vi "CreateRequests.vi"(8 "error in (no error)":errorcluster) -> (0 "error out":errorcluster, 3 "StandardRequests":T1)   [LabVIEW 2024, in "Module.lvclass"]
uses:
  Module.lvclass
  Module.lvclass/Module.ctl
  StopEventArgs.ctl
  StandardRequests.ctl
  Show Front Panel--Args.ctl
  Hide Front Panel.ctl
  Show Block Diagram.ctl
  Hide Block Diagram--Args.ctl
  InitialiseArgs.ctl
  Reply.ctl
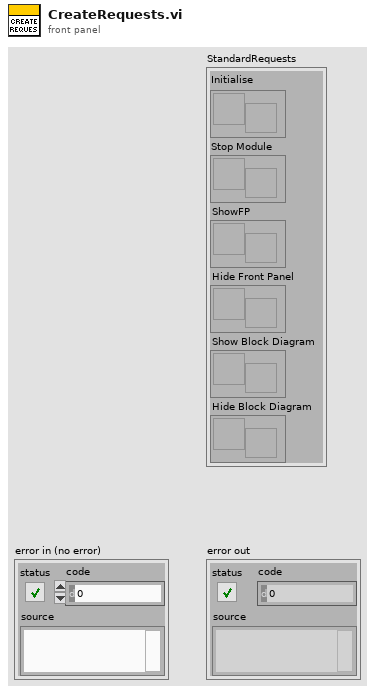
[diagram p1: front panel]
types:
  T1 = typedef "Module.lvclass/StandardRequests.ctl" = cluster{"Initialise":refnum<user-event>, "Stop Module":refnum<user-event>, "ShowFP":refnum<user-event>, "Hide Front Panel":refnum<user-event>, "Show Block Diagram":refnum<user-event>, "Hide Block Diagram":refnum<user-event>}
  T2 = typedef "Module.lvclass/InitialiseArgs.ctl" = cluster{"null":bool}
  T3 = typedef "Module.lvclass/Reply.ctl" = cluster{"Expects Reply":bool, "Reply":refnum<notifier>}
  T4 = typedef "Module.lvclass/Hide Block Diagram--Args.ctl" = bool
  T5 = typedef "Module.lvclass/Show Block Diagram.ctl" = bool
  T6 = typedef "Module.lvclass/Hide Front Panel.ctl" = variant
  T7 = typedef "Module.lvclass/Show Front Panel--Args.ctl" = variant
  T8 = typedef "Module.lvclass/StopEventArgs.ctl" = bool
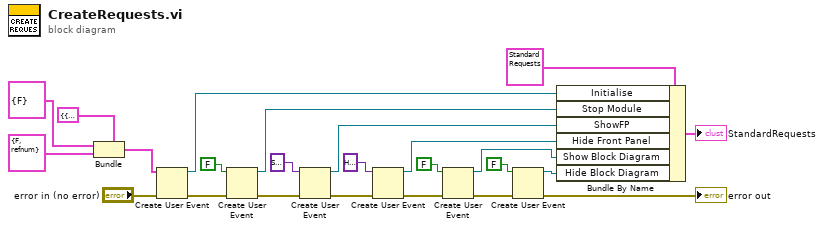
[diagram p0: block diagram]
diagram:
  n1 = Bundle(cluster=cluster{"Args":T2, "Reply":T3} {"Args"={"null"=FALSE}, "Reply"={"Expects Reply"=FALSE, "Reply"=refnum}} ("Message"), "Args"=T2 {"null"=FALSE}, "Reply"=T3 {"Expects Reply"=FALSE, "Reply"=refnum}) -> (w5:cluster{"Args":T2, "Reply":T3})
  n2 = Create User Event(user event datatype=w5, error in="error in (no error)") -> (user event=w4:refnum<user-event>, error out=w1:errorcluster)
  n3 = Create User Event(user event datatype=T8 FALSE ("Stop"), error in=w1) -> (user event=w23:refnum<user-event>, error out=w20:errorcluster)
  n4 = Create User Event(user event datatype=T7 variant ("Data"), error in=w20) -> (user event=w18:refnum<user-event>, error out=w15:errorcluster)
  n5 = Create User Event(user event datatype=T6 variant ("Data"), error in=w15) -> (user event=w13:refnum<user-event>, error out=w16:errorcluster)
  n6 = Create User Event(user event datatype=T5 FALSE ("Data 2"), error in=w16) -> (user event=w12:refnum<user-event>, error out=w9:errorcluster)
  n7 = Create User Event(user event datatype=T4 FALSE ("null"), error in=w9) -> (user event=w10:refnum<user-event>, error out=→"error out":errorcluster)
  n8 = Bundle By Name(cluster=T1 {"Initialise"=refnum, "Stop Module"=refnum, "ShowFP"=refnum, "Hide Front Panel"=refnum, "Show Block Diagram"=refnum, "Hide Block Diagram"=refnum} ("StandardEvents"), "Initialise"=w4, "Stop Module"=w23, "ShowFP"=w18, "Hide Front Panel"=w13, "Show Block Diagram"=w12, "Hide Block Diagram"=w10) -> (→"StandardRequests":T1)
